vi "Manual Test.vi"() -> ()   [LabVIEW 2020, in "ChromTech MX-Class Drivers.lvlib"]
uses:
  <instrlib>/RxnRover/ChromtechNextGenDriver/ChromTech MX-Class Drivers.lvlib
panel:
  in  "Retry Attempts":i32
  out "error out":errorcluster
  in  "Stop Pump":bool
  in  "Start Pump":bool
  in  "Get User Compensation":bool
  out "Current User Compensation":dbl
  in  "stop":bool
  in  "error in (no error)":errorcluster
  in  "Fast Comms":bool
  in  "Get Current Status":bool
  out "Pressure Units":string
  out "Lower Pressure Limit":dbl
  out "Upper Pressure Limit":dbl
  in  "Get Maximum Flow Rate":bool
  out "Maximum Flow Rate":dbl
  in  "Get Pump Information":bool
  out "Lower Pressure Fault":bool
  out "Motor Stall":bool
  out "Keypad Enabled":bool
  out "Upper Pressure Fault":bool
  out "In Prime":bool
  out "Running":bool
  out "Head Identifier":string
  out "Pressure Compensation":i32
  out "Current Flow Rate":dbl
  out "Current Pressure":dbl
  in  "Get Current Conditions":bool
  in  "Get Firmware Details":bool
  out "Firmware Version":string
  out "Firmware Part Number":dbl
  in  "Set User Comp":bool
  in  "User Compensation":dbl=100.0
  in  "VISA resource name":refnum<visa-resource-name>
  in  "Set Flow Rate":bool
  in  "Flow Rate":dbl
  # "Teledyne SSI MX-Class Pump"
  # "Set Conditions"
  # "Current Status"
  # "Firmware Information"
  # "Still Under constuction. Should probably be reworked into state machine and \nexplicitly make a test button for each driver VI."
  # "Get Conditions"
  # "Pump Information"
  # "Pump Control"
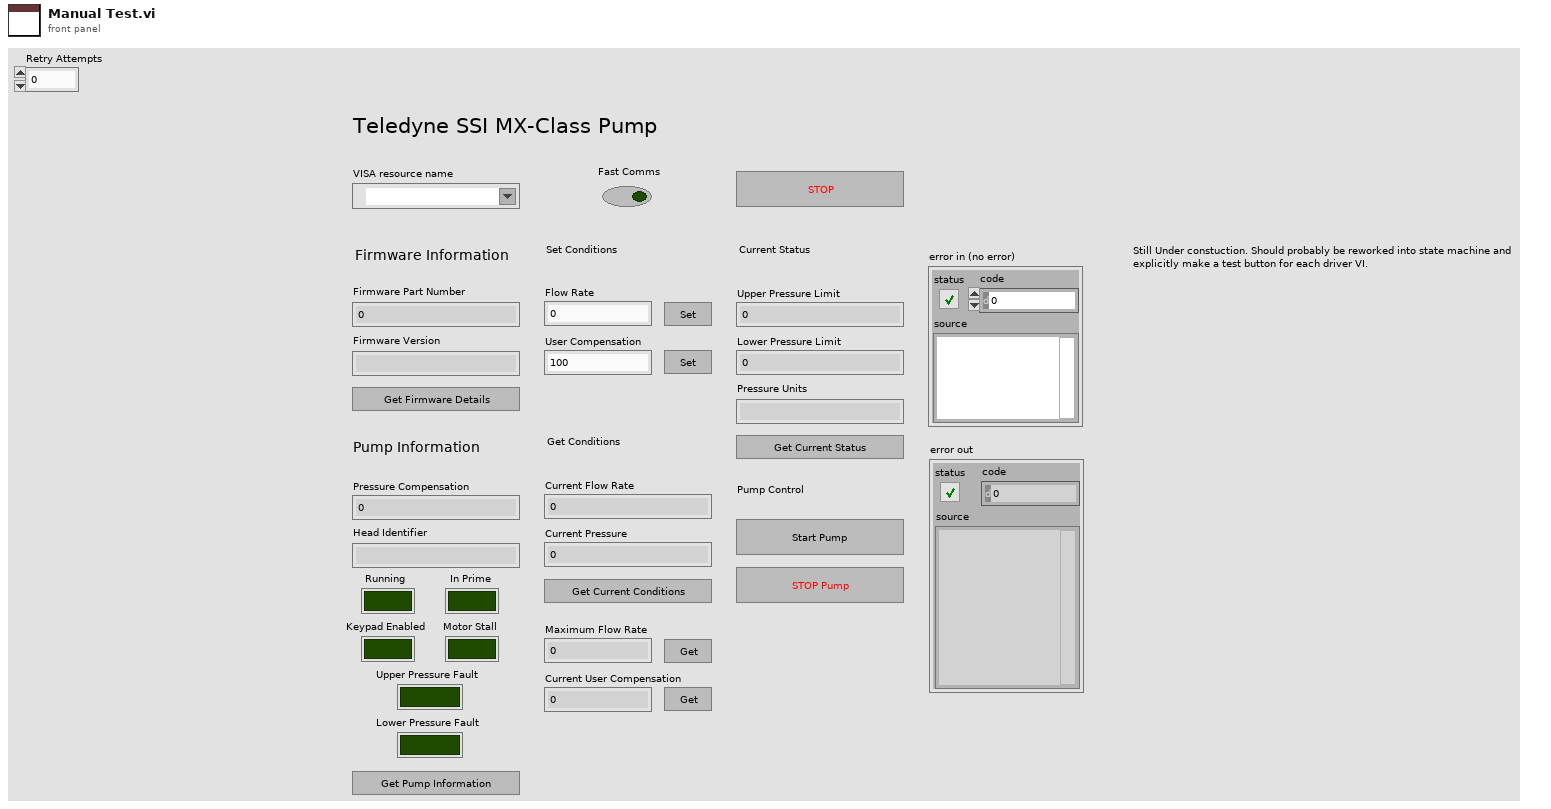
[diagram p1: front panel]
types:
  T1 = cluster{"Baud Rate":u32, "Parity":u16, "Flow Control":u16, "Data Bits":u16, "Stop Bits":u16}
  T2 = cluster{"Flow rate":dbl, "Running":bool, "Pressure Comp":i32, "Head ID":string, "Upper Pressure Fault":bool, "Lower Pressure Fault":bool, "In Prime":bool, "Keypad Enabled":bool, "Motor Stall Fault":bool}
  T3 = cluster{"Flow rate":dbl, "Upper Pressure Limit":dbl, "Lower Pressure Limit":dbl, "Pressure Units":string, "Running?":bool}
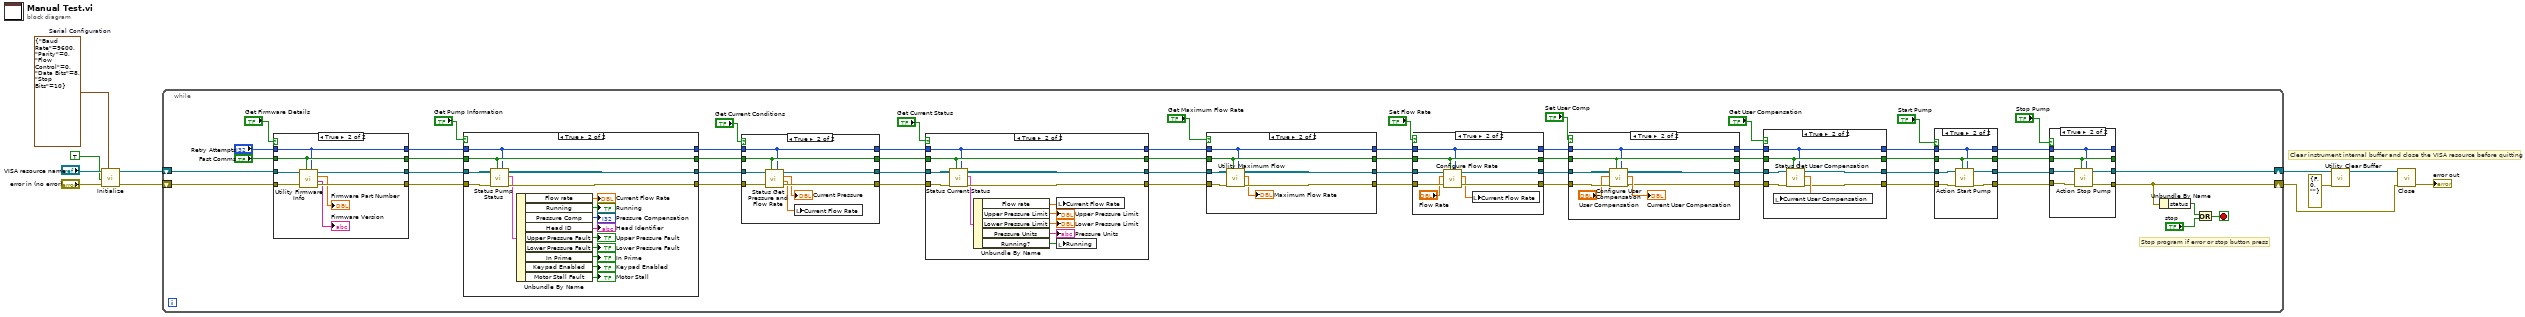
[diagram p0: block diagram]
diagram:
  w6 = T1 {"Baud Rate"=9600, "Parity"=0, "Flow Control"=0, "Data Bits"=8, "Stop Bits"=10}  # Serial Configuration
  # "Clear instrument internal buffer and close the VISA resource before quitting"
  n1 = call <instrlib>:"Initialize.vi"("Serial Configuration"=w6, "error in (no error)"="error in (no error)", "Fast Comms (F)"=TRUE, "VISA resource name"="VISA resource name") -> ("error out"=w8:errorcluster, "VISA resource name out"=w10:refnum<visa-resource-name>)  [unwired: 6 in]
  n2 = while {
    shift-right: [w22] -> w1
    shift-left: w8 -> [w54]
    shift-right: [w23] -> w3
    shift-left: w10 -> [w42]
    stop <- w26 stop-if-true
    # "Stop program if error or stop button press"
    n3 = case shown="True" "Get Firmware Details" {
      tunnel: w42 -> [w172 w180]
      tunnel: w54 -> [w171 w179]
      tunnel: [w172 w178] -> w45
      tunnel: [w171 w177] -> w41
      tunnel: [w170 w174] -> w53
      tunnel: "Fast Comms" -> [w170 w174]
      tunnel: "Retry Attempts" -> [w169 w173]
      tunnel: [w169 w173] -> w20
      frame False {
      }
      frame True {
        n4 = call <instrlib>:"Utility Firmware Info.vi"("Retry Attempts (0)"=w173, "Fast Comms (F)"=w174, "error in"=w179, "VISA resource name"=w180) -> ("error out"=w177:errorcluster, "Firmware Version"=→"Firmware Version":string, "Firmware Part Number"=→"Firmware Part Number":dbl, "VISA resource name out"=w178:refnum<visa-resource-name>)  [unwired: 4 in]
      }
    }
    n5 = case shown="True" "Get Pump Information" {
      tunnel: w45 -> [w153 w168]
      tunnel: [w153 w167] -> _
      tunnel: w41 -> [w152 w166]
      tunnel: [w152 w166] -> w40
      tunnel: w53 -> [w151 w155]
      tunnel: [w151 w155] -> w46
      tunnel: w20 -> [w150 w154]
      tunnel: [w150 w154] -> w19
      frame False {
      }
      frame True {
        n6 = call <instrlib>:"Status Pump Status.vi"("Retry Attempts (0)"=w154, "Fast Comms (F)"=w155, "error in (no error)"=w166, "VISA resource name"=w168) -> ("Status Cluster"=w165:T2, "VISA resource name out"=w167:refnum<visa-resource-name>)  [unwired: 5 in, 1 out]
        n7 = Unbundle By Name(w165) -> ("Flow rate"=→"Current Flow Rate":dbl, "Running"=→"Running":bool, "Pressure Comp"=→"Pressure Compensation":i32, "Head ID"=→"Head Identifier":string, "Upper Pressure Fault"=→"Upper Pressure Fault":bool, "Lower Pressure Fault"=→"Lower Pressure Fault":bool, "In Prime"=→"In Prime":bool, "Keypad Enabled"=→"Keypad Enabled":bool, "Motor Stall Fault"=→"Motor Stall":bool)
      }
    }
    n8 = case shown="True" "Get Current Conditions" {
      tunnel: w45 -> [w140 w149]
      tunnel: [w140 w148] -> _
      tunnel: w40 -> [w139 w147]
      tunnel: [w139 w146] -> w39
      tunnel: w46 -> [w141 w143]
      tunnel: [w141 w143] -> _
      tunnel: w19 -> [w138 w142]
      tunnel: [w138 w142] -> w18
      frame False {
      }
      frame True {
        n9 = call <instrlib>:"Status Get Pressure and Flow Rate.vi"("Retry Attempts (0)"=w142, "Fast Comms (F)"=w143, "error in"=w147, "VISA resource name"=w149) -> ("error out"=w146:errorcluster, "Flow Rate"=w144:dbl, "Pressure"=→"Current Pressure":dbl, "VISA resource name out"=w148:refnum<visa-resource-name>)  [unwired: 4 in]
        n10 = local write "Current Flow Rate"(w144) -> ()
      }
    }
    n11 = case shown="True" "Get Current Status" {
      tunnel: w46 -> [w123 w127]
      tunnel: [w123 w127] -> _
      tunnel: w45 -> [w124 w137]
      tunnel: [w124 w136] -> _
      tunnel: w39 -> [w125 w135]
      tunnel: [w125 w134] -> w38
      tunnel: w18 -> [w122 w126]
      tunnel: [w122 w126] -> w17
      frame False {
      }
      frame True {
        n12 = call <instrlib>:"Status Current Status.vi"("Retry Attempts (0)"=w126, "Fast Comms (F)"=w127, "error in (no error)"=w135, "VISA resource name"=w137) -> ("error out"=w134:errorcluster, "Status Cluster"=w133:T3, "VISA resource name out"=w136:refnum<visa-resource-name>)  [unwired: 5 in]
        n13 = Unbundle By Name(w133) -> ("Flow rate"=w132:dbl, "Upper Pressure Limit"=→"Upper Pressure Limit":dbl, "Lower Pressure Limit"=→"Lower Pressure Limit":dbl, "Pressure Units"=→"Pressure Units":string, "Running?"=w128:bool)
        n14 = local write "Current Flow Rate"(w132) -> ()
        n15 = local write "Running"(w128) -> ()
      }
    }
    n16 = case shown="True" "Get Maximum Flow Rate" {
      tunnel: w45 -> [w113 w121]
      tunnel: w38 -> [w112 w119]
      tunnel: [w113 w120] -> _
      tunnel: w46 -> [w114 w116]
      tunnel: [w114 w116] -> _
      tunnel: [w112 w118] -> w37
      tunnel: w17 -> [w111 w115]
      tunnel: [w111 w115] -> w16
      frame False {
      }
      frame True {
        n17 = call <instrlib>:"Utility Maximum Flow.vi"("Retry Attempts (0)"=w115, "Fast Comms (F)"=w116, "error in"=w119, "VISA resource name"=w121) -> ("error out"=w118:errorcluster, "Maximum Flow"=→"Maximum Flow Rate":dbl, "VISA resource name out"=w120:refnum<visa-resource-name>)  [unwired: 5 in]
      }
    }
    n18 = case shown="True" "Set Flow Rate" {
      tunnel: w46 -> [w102 w104]
      tunnel: w45 -> [w101 w110]
      tunnel: w37 -> [w100 w108]
      tunnel: [w102 w104] -> _
      tunnel: [w101 w109] -> _
      tunnel: [w100 w107] -> w36
      tunnel: w16 -> [w99 w103]
      tunnel: [w99 w103] -> w15
      frame False {
      }
      frame True {
        n19 = call <instrlib>:"Configure Flow Rate.vi"("Retry Attempts (0)"=w103, "Fast Comms (F)"=w104, "error in"=w108, "Flow Input (ml/min)"="Flow Rate", "VISA resource name"=w110) -> ("error out"=w107:errorcluster, "Flow Output"=w105:dbl, "VISA resource name out"=w109:refnum<visa-resource-name>)  [unwired: 4 in]
        n20 = local write "Current Flow Rate"(w105) -> ()
      }
    }
    n21 = case shown="True" "Set User Comp" {
      tunnel: w46 -> [w90 w92]
      tunnel: w45 -> [w89 w98]
      tunnel: w36 -> [w88 w96]
      tunnel: [w90 w92] -> _
      tunnel: [w89 w97] -> _
      tunnel: [w88 w93] -> w35
      tunnel: w15 -> [w87 w91]
      tunnel: [w87 w91] -> w14
      frame False {
      }
      frame True {
        n22 = call <instrlib>:"Configure User Compensation.vi"("Retry Attempts (0)"=w91, "Fast Comms (F)"=w92, "error in"=w96, "Compensation (%)"="User Compensation", "VISA resource name"=w98) -> ("error out"=w93:errorcluster, "Response Compensation"=→"Current User Compensation":dbl, "VISA resource name out"=w97:refnum<visa-resource-name>)  [unwired: 4 in]
      }
    }
    n23 = case shown="True" "Get User Compensation" {
      tunnel: w46 -> [w79 w81]
      tunnel: w45 -> [w78 w86]
      tunnel: w35 -> [w77 w84]
      tunnel: [w77 w82] -> w32
      tunnel: [w78 w85] -> w33
      tunnel: [w79 w81] -> w28
      tunnel: w14 -> [w76 w80]
      tunnel: [w76 w80] -> w13
      frame False {
      }
      frame True {
        n24 = call <instrlib>:"Status Get User Compensation.vi"("Retry Attempts (0)"=w80, "Fast Comms (F)"=w81, "error in"=w84, "VISA resource name"=w86) -> ("error out"=w82:errorcluster, "User Compensation"=w83:dbl, "VISA resource name out"=w85:refnum<visa-resource-name>)  [unwired: 5 in]
        n25 = local write "Current User Compensation"(w83) -> ()
      }
    }
    n26 = case shown="True" "Start Pump" {
      tunnel: [w69 w73] -> w30
      tunnel: w33 -> [w69 w74]
      tunnel: [w68 w72] -> w29
      tunnel: w32 -> [w68 w75]
      tunnel: [w67 w71] -> w27
      tunnel: w28 -> [w67 w71]
      tunnel: w13 -> [w66 w70]
      tunnel: [w66 w70] -> w12
      frame False {
      }
      frame True {
        n27 = call <instrlib>:"Action Start Pump.vi"("Retry Attempts (0)"=w70, "Fast Comms (F)"=w71, "error in"=w75, "VISA resource name"=w74) -> ("error out"=w72:errorcluster, "VISA resource name out"=w73:refnum<visa-resource-name>)  [unwired: 6 in]
      }
    }
    n28 = case shown="True" "Stop Pump" {
      tunnel: [w59 w63] -> w23
      tunnel: w30 -> [w59 w64]
      tunnel: [w58 w62] -> w22
      tunnel: w29 -> [w58 w65]
      tunnel: w27 -> [w57 w61]
      tunnel: [w57 w61] -> _
      tunnel: w12 -> [w56 w60]
      tunnel: [w56 w60] -> _
      frame False {
      }
      frame True {
        n29 = call <instrlib>:"Action Stop Pump.vi"("Retry Attempts (0)"=w60, "Fast Comms (F)"=w61, "error in"=w65, "VISA resource name"=w64) -> ("error out"=w62:errorcluster, "VISA resource name out"=w63:refnum<visa-resource-name>)  [unwired: 6 in]
      }
    }
    n30 = Unbundle By Name(w22) -> ("status"=w25:bool)
    n31 = Or(x=w25, y="stop") -> (x .or. y?=w26:bool)
  }
  n32 = call <instrlib>:"Utility Clear Buffer.vi"("error in (no error)"=errorcluster {"status"=FALSE, "code"=0, "source"=""}, "VISA resource name"=w3) -> ("VISA resource name out"=w5:refnum<visa-resource-name>)  [unwired: 8 in, 1 out]
  n33 = call <instrlib>:"Close.vi"("error in (no error)"=w1, "VISA resource name"=w5) -> ("error out"=→"error out":errorcluster)  [unwired: 9 in]
